vi "Servo Scanner with limits.vi"() -> ()   [LabVIEW 2016]
panel:
  in  "stop":bool
  out "x2":dbl
  out "x":dbl
  out "Up or Down":bool
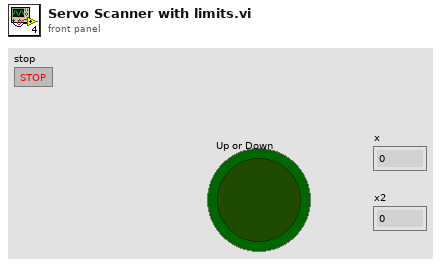
[diagram p1: front panel]
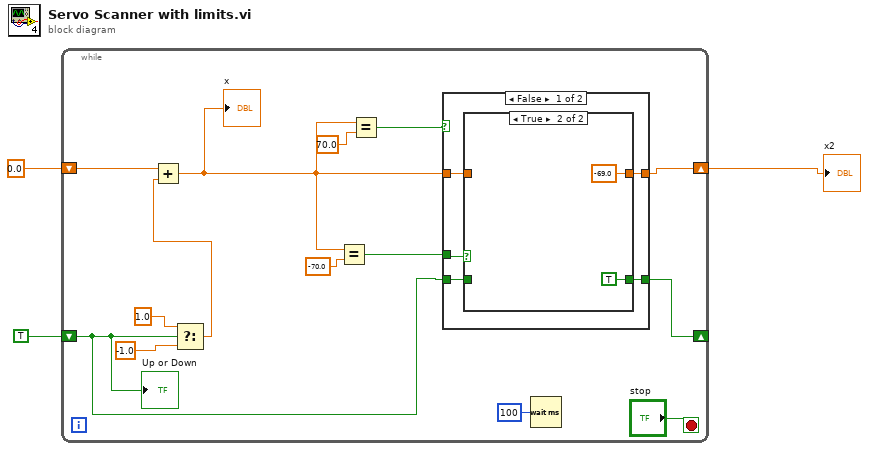
[diagram p0: block diagram]
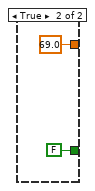
[diagram p3: hidden frame]
diagram:
  n1 = while {
    shift-right: [w7] -> w1
    shift-left: 0.0 ("x") -> [w15]
    shift-right: [w5] -> _
    shift-left: TRUE ("Up or Down") -> [w6]
    stop <- "stop" stop-if-true
    n2 = Select(t=1.0, s=w6, f=-1.0) -> (s? t:f=w12:dbl)
    n3 = Add(x=w15, y=w12) -> (x+y=w4:dbl)
    "x" <- w4
    n4 = Equal?(x=w4, y=-70.0) -> (x = y?=w8:bool)
    n5 = Equal?(x=w4, y=70.0) -> (x = y?=w9:bool)
    n6 = case shown="False" w9 {
      tunnel: w8 -> [w22 _]
      tunnel: w4 -> [w21 _]
      tunnel: [w20 69.0] -> w7
      tunnel: w6 -> [w19 _]
      tunnel: [w18 FALSE ("Up or Down")] -> w5
      frame False {
        n7 = case shown="True" w22 {
          tunnel: w21 -> [w24 _]
          tunnel: [w24 -69.0] -> w20
          tunnel: w19 -> [w23 _]
          tunnel: [w23 TRUE ("Up or Down")] -> w18
          frame False {
          }
          frame True {
          }
        }
      }
      frame True {
      }
    }
    n8 = Wait (ms)(milliseconds to wait=u32 100) -> ()  [unwired: 1 out]
    "Up or Down" <- w6
  }
  "x2" <- w1
